vi "ComputeACPadPositions.vi"(0 "Theta Calibration":dbl format="%#_10g", 1 "X cp":dbl format="%#_10g", 2 "Y cp":dbl format="%#_10g", 3 "Stage Initial\nRotation":dbl, 4 "Sensor Path":path=path "R0Hamamatsu.txt ") -> ()   [LabVIEW 2018]
uses:
  <vilib>/Analysis/coordinate.llb/2D Cartesian Coordinate Rotation (Scalar).vi
  <vilib>/Utility/file.llb/Read Delimited Spreadsheet (DBL).vi
  <vilib>/Utility/file.llb/Write Delimited Spreadsheet (DBL).vi
  <vilib>/Analysis/NI_AALPro.lvlib
panel:
  out "error out":errorcluster
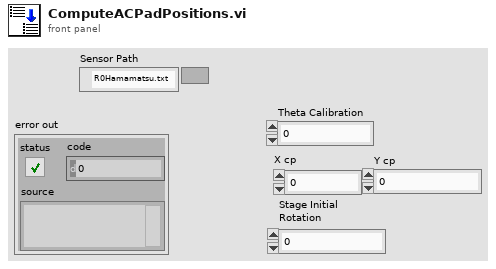
[diagram p1: front panel]
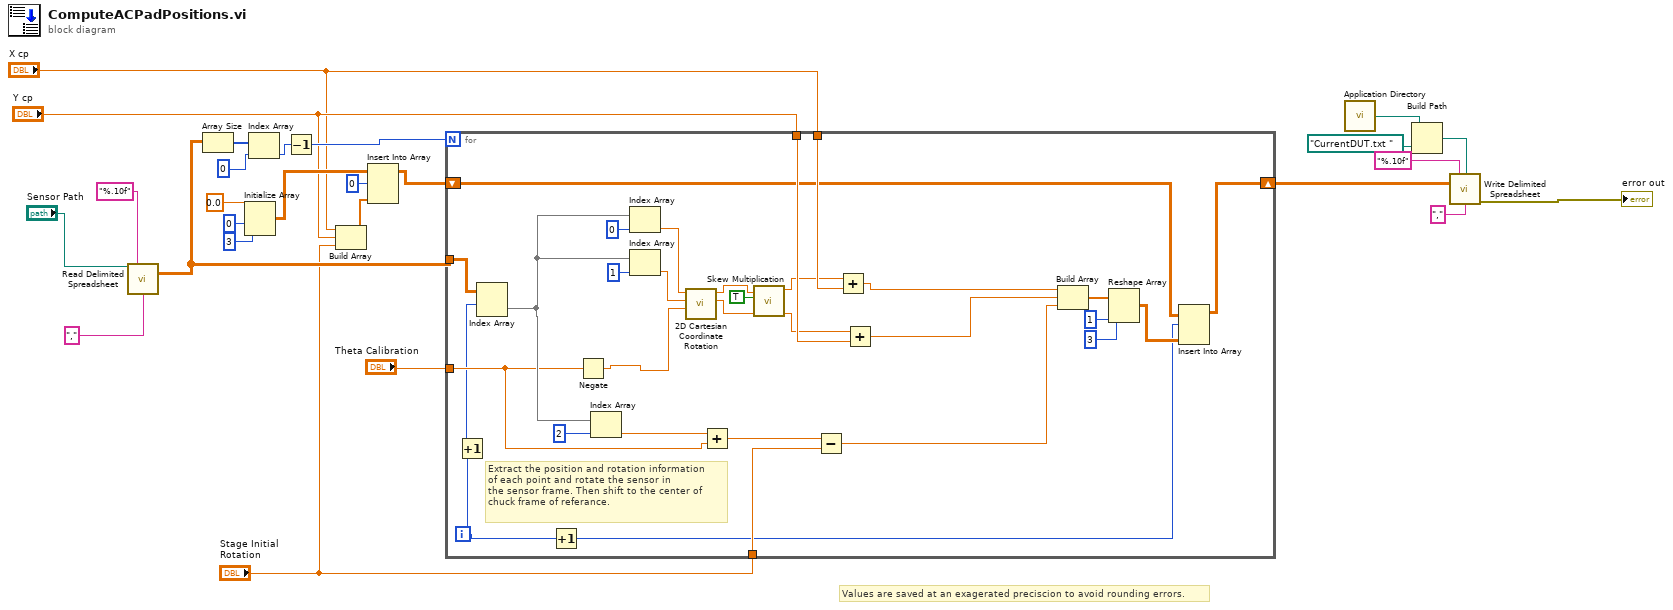
[diagram p0: block diagram]
diagram:
  # "Values are saved at an exagerated preciscion to avoid rounding errors."
  n1 = call-poly <vilib>:"Read Delimited Spreadsheet.vi"("file path (dialog if empty)"="Sensor Path", "format (%.3f)"="%.10f", "delimiter (\\t)"="," ("delimiter (\\t)")) -> ("all rows"=w23:dbl[][])  [unwired: 7 in, 5 out]
  n2 = Array Size(array=w23) -> (size(s)=w25:i32[])
  n3 = Initialize Array(0.0 ("element"), 0 ("dimension size"), 3 ("dimension size")) -> (w7:dbl[][])
  n4 = Index Array(array=w25, index=0) -> (element=w22:i32)
  n5 = Decrement(x=w22) -> (x-1=w9:i32)
  n6 = Build Array("X cp", "Y cp", "Stage Initial\nRotation") -> (w2:dbl[])
  n7 = Insert Into Array(array=w7, index (row)=0, new element=w2) -> (w8:dbl[][])  [unwired: 1 in]
  n8 = for {
    N: w9 -> [_]
    tunnel: w23 -> [w57]
    tunnel: "Theta Calibration" -> [w49]
    tunnel: "X cp" -> [w52]
    tunnel: "Y cp" -> [w51]
    tunnel: "Stage Initial\nRotation" -> [w30]
    shift-right: [w44] -> w15
    shift-left: w8 -> [w45]
    i -> [w42]
    # "Extract the position and rotation information \nof each point and rotate the sensor in \nthe sensor frame. Then shift to the center of \nchuck frame of referance."
    n9 = Increment(x=w42) -> (x+1=w38:i32)
    n10 = Index Array(array=w57, index (row)=w38) -> (element=w56:dbl[])  [unwired: 1 in]
    n11 = Increment(x=w42) -> (x+1=w27:i32)
    n12 = Negate(x=w49) -> (-x=w31:dbl)
    n13 = Index Array(array=w56, index=2) -> (element=w50:dbl)
    n14 = Index Array(array=w56, index=0) -> (element=w41:dbl)
    n15 = Index Array(array=w56, index=1) -> (element=w40:dbl)
    n16 = call-poly <vilib>:"2D Cartesian Coordinate Rotation.vi"("theta"=w31, "y"=w40, "x"=w41) -> ("y out"=w35:dbl, "x out"=w34:dbl)  [unwired: 6 in, 1 out]
    n17 = Add(x=w50, y=w49) -> (x+y=w29:dbl)
    n18 = call "Skew Multiplication.vi"("Y"=w35, "Boolean"=TRUE, "X"=w34) -> ("Y'"=w32:dbl, "X'"=w33:dbl)  [unwired: 7 in]
    n19 = Subtract(x=w29, y=w30) -> (x-y=w28:dbl)
    n20 = Add(x=w33, y=w52) -> (x+y=w37:dbl)
    n21 = Add(x=w32, y=w51) -> (x+y=w36:dbl)
    n22 = Build Array(w37, w36, w28) -> (w48:dbl[])
    n23 = Reshape Array(w48, 1 ("dimension size"), 3 ("dimension size")) -> (w43:dbl[][])
    n24 = Insert Into Array(array=w45, index (row)=w27, new element=w43) -> (w44:dbl[][])  [unwired: 1 in]
  }
  n25 = call <vilib>:"Application Directory.vi"() -> ("Application Directory"=w17:path)
  n26 = Build Path(base path=w17, name or relative path=path "CurrentDUT.txt " ("file path (dialog if empty)")) -> (appended path=w16:path)
  n27 = call-poly <vilib>:"Write Delimited Spreadsheet.vi"("file path (dialog if empty)"=w16, "format (%.3f)"="%.10f", "2D data"=w15, "delimiter (\\t)"="," ("delimiter (\\t)")) -> ("error out"=→"error out":errorcluster)  [unwired: 10 in, 1 out]
